vi "MultiChannelExample.vi"() -> ()   [LabVIEW 2020]
uses:
  PalmSens/PalmSens.lvclass
  D:/PalmSensAppsAndSDKS/LabVIEW/PalmSens SDK for LabVIEW 5.10/PalmSens/Libraries/PalmSens.Core.dll
  PalmSens/Libraries/PalmSens.Core.dll
  PalmSens/MeasurementsResult.ctl
  PalmSens/MeasurementResults.ctl
  PalmSens/LiveCurveResult.ctl
panel:
  out "Measurements":T1
  out "Array 2":string[](array[string])
  out "Is Measuring 2":bool
  in  "PalmSens.lvclass 2":refnum<class "PalmSens.lvclass">
  out "LSV Method Indicator":refnum<k24>
  out "Array":string[](array[string])
  out "Is Measuring":bool
  in  "PalmSens.lvclass":refnum<class "PalmSens.lvclass">
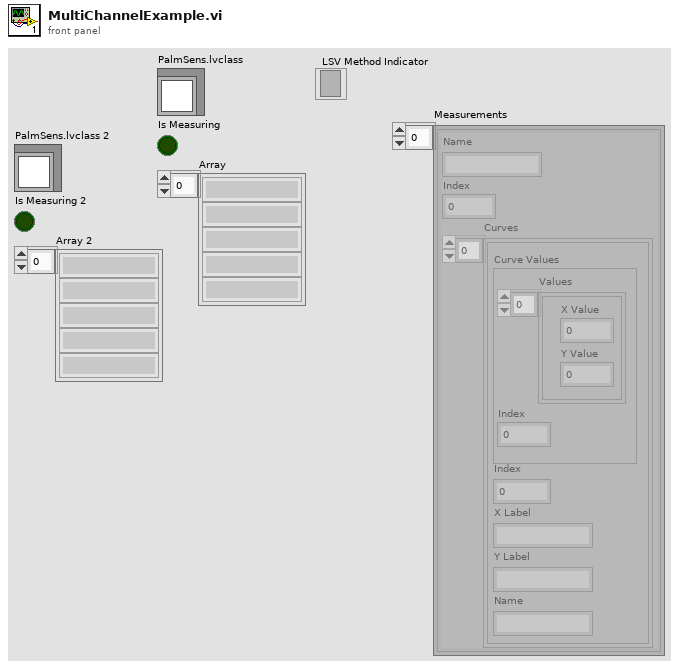
[diagram p1: front panel]
types:
  T1 = typedef "MeasurementsResult.ctl" = cluster{"Name":string, "Curves":T2, "Index":i32}[]
  T2 = typedef "MeasurementResults.ctl" = T3[]
  T3 = typedef "LiveCurveResult.ctl" = cluster{"X Label":string, "Y Label":string, "Name":string, "Index":i16, "Curve Values":cluster{"Values":cluster{"X Value":dbl, "Y Value":dbl}[], "Index":i16}}
  T4 = cluster{"Active Measurement":refnum<k24>, "Is Measuring Refnum":refnum<vi>, "Live Curve Result Refnum":refnum<vi>}
  T5 = cluster{"Active Measurement":refnum<k24>, "Is Measuring Refnum":refnum<vi>, "Live Curve Result Refnum":refnum<vi>}[]
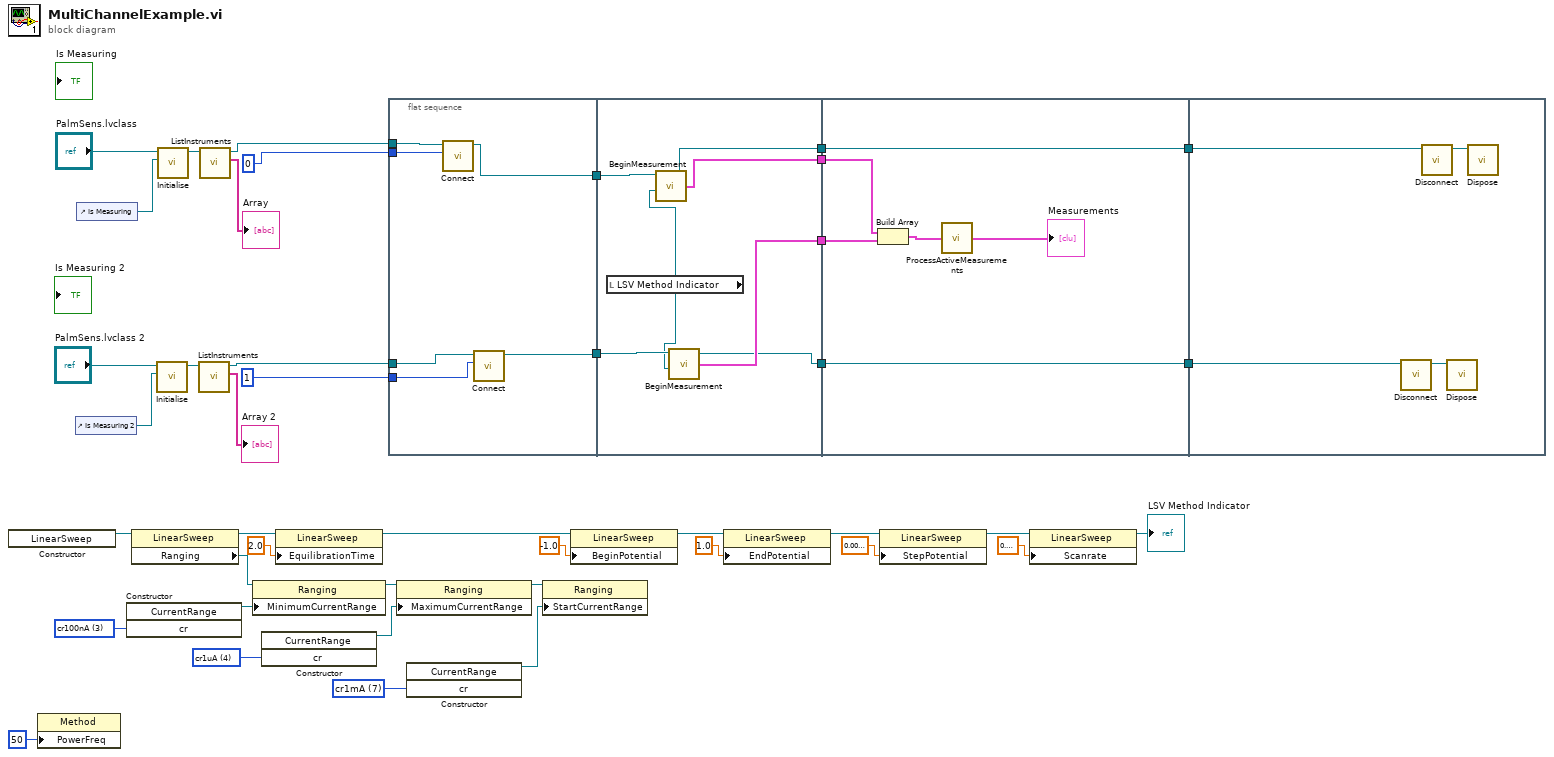
[diagram p0: block diagram]
diagram:
  w31 = 4 items=["cr100pA"=0, "cr1nA"=1, "cr10nA"=2, "cr100nA"=3, "cr1uA"=4, "cr10uA"=5, "cr100uA"=6, "cr1mA"=7, "cr10mA"=8, "cr100mA"=9, "cr2uA"=10, "cr4uA"=11, "cr8uA"=12, "cr16uA"=13, "cr32uA"=14, "cr125uA"=17, "cr250uA"=18, "cr500uA"=19, "cr5mA"=20, "cr6uA"=21, "cr13uA"=22, "cr25uA"=23, "cr50uA"=24, "cr200uA"=25, "cr63uA"=26] ("cr")
  w32 = 7 items=["cr100pA"=0, "cr1nA"=1, "cr10nA"=2, "cr100nA"=3, "cr1uA"=4, "cr10uA"=5, "cr100uA"=6, "cr1mA"=7, "cr10mA"=8, "cr100mA"=9, "cr2uA"=10, "cr4uA"=11, "cr8uA"=12, "cr16uA"=13, "cr32uA"=14, "cr125uA"=17, "cr250uA"=18, "cr500uA"=19, "cr5mA"=20, "cr6uA"=21, "cr13uA"=22, "cr25uA"=23, "cr50uA"=24, "cr200uA"=25, "cr63uA"=26] ("cr")
  w36 = 3 items=["cr100pA"=0, "cr1nA"=1, "cr10nA"=2, "cr100nA"=3, "cr1uA"=4, "cr10uA"=5, "cr100uA"=6, "cr1mA"=7, "cr10mA"=8, "cr100mA"=9, "cr2uA"=10, "cr4uA"=11, "cr8uA"=12, "cr16uA"=13, "cr32uA"=14, "cr125uA"=17, "cr250uA"=18, "cr500uA"=19, "cr5mA"=20, "cr6uA"=21, "cr13uA"=22, "cr25uA"=23, "cr50uA"=24, "cr200uA"=25, "cr63uA"=26] ("cr")
  n1 = constructor class="LinearSweep"() -> (reference out=w38:refnum<k24>)  [unwired: 3 in, 2 out]
  n2 = property class="Method"("PowerFreq"=50) -> ()  [unwired: 2 in, 2 out]
  n3 = control-ref of="Is Measuring 2"() -> (w15:refnum<vi>)
  n4 = control-ref of="Is Measuring"() -> (w41:refnum<vi>)
  n5 = constructor class="CurrentRange"("cr"=w36) -> (reference out=w35:refnum<k24>)  [unwired: 3 in, 3 out]
  n6 = property class="LinearSweep"(reference=w38) -> (reference out=w28:refnum<k24>, "Ranging"=w37:refnum<k24>)  [unwired: 1 in, 1 out]
  n7 = call-dynamic "Initialise.vi"("Is Measuring Refnum"=w15, "PalmSens in"="PalmSens.lvclass 2") -> ("PalmSens out"=w14:refnum<class "PalmSens.lvclass">)  [unwired: 8 in, 1 out]
  n8 = call-dynamic "Initialise.vi"("Is Measuring Refnum"=w41, "PalmSens in"="PalmSens.lvclass") -> ("PalmSens out"=w40:refnum<class "PalmSens.lvclass">)  [unwired: 8 in, 1 out]
  n9 = call-dynamic "ListInstruments.vi"("PalmSens in"=w14) -> ("Array"=→"Array 2":string[], "PalmSens out"=w1:refnum<class "PalmSens.lvclass">)  [unwired: 8 in, 1 out]
  n10 = call-dynamic "ListInstruments.vi"("PalmSens in"=w40) -> ("Array"=→"Array":string[], "PalmSens out"=w3:refnum<class "PalmSens.lvclass">)  [unwired: 8 in, 1 out]
  n11 = property class="Ranging"(reference=w37, "MinimumCurrentRange"=w35) -> (reference out=w34:refnum<k24>)  [unwired: 1 in, 1 out]
  n12 = constructor class="CurrentRange"("cr"=w31) -> (reference out=w29:refnum<k24>)  [unwired: 3 in, 3 out]
  n13 = property class="LinearSweep"(reference=w28, "EquilibrationTime"=sgl 2.0) -> (reference out=w26:refnum<k24>)  [unwired: 1 in, 1 out]
  n14 = flat-sequence {
    tunnel: [w46] -> w6
    tunnel: [w43] -> w5
    tunnel: 0 ("Instrument Index") -> [w48]
    tunnel: w3 -> [w47]
    tunnel: 1 ("Instrument Index") -> [w45]
    tunnel: w1 -> [w44]
    tunnel: [w53] -> w10
    tunnel: [w50] -> w9
    tunnel: [w54] -> w8
    tunnel: [w51] -> w7
    tunnel: w6 -> [w55]
    tunnel: w5 -> [w52]
    tunnel: [w61] -> w12
    tunnel: [w60] -> w11
    tunnel: w10 -> [w61]
    tunnel: w9 -> [w60]
    tunnel: w8 -> [w59]
    tunnel: w7 -> [w58]
    tunnel: w12 -> [w63]
    tunnel: w11 -> [w62]
    frame #0 {
      n15 = call-dynamic "Connect.vi"("Instrument Index"=w48, "PalmSens in"=w47) -> ("PalmSens out"=w46:refnum<class "PalmSens.lvclass">)  [unwired: 8 in, 1 out]
      n16 = call-dynamic "Connect.vi"("Instrument Index"=w45, "PalmSens in"=w44) -> ("PalmSens out"=w43:refnum<class "PalmSens.lvclass">)  [unwired: 8 in, 1 out]
    }
    frame #1 {
      n17 = local read "LSV Method Indicator"() -> (w49:refnum<k24>)
      n18 = call-dynamic "BeginMeasurement.vi"("Method .NET Refnum"=w49, "PalmSens in"=w55) -> ("Active Measurement Info"=w54:T4, "PalmSens out"=w53:refnum<class "PalmSens.lvclass">)  [unwired: 2 in, 1 out]
      n19 = call-dynamic "BeginMeasurement.vi"("Method .NET Refnum"=w49, "PalmSens in"=w52) -> ("Active Measurement Info"=w51:T4, "PalmSens out"=w50:refnum<class "PalmSens.lvclass">)  [unwired: 2 in, 1 out]
    }
    frame #2 {
      n20 = Build Array(w59, w58) -> (w57:T5)
      n21 = call "ProcessActiveMeasurements.vi"("Active Measurements"=w57) -> ("Measurements"=→"Measurements":T1)
    }
    frame #3 {
      n22 = call-dynamic "Disconnect.vi"("PalmSens in"=w62) -> ("PalmSens out"=w64:refnum<class "PalmSens.lvclass">)  [unwired: 9 in, 1 out]
      n23 = call-dynamic "Disconnect.vi"("PalmSens in"=w63) -> ("PalmSens out"=w65:refnum<class "PalmSens.lvclass">)  [unwired: 9 in, 1 out]
      n24 = call-dynamic "Dispose.vi"("PalmSens in"=w64) -> ()  [unwired: 9 in, 2 out]
      n25 = call-dynamic "Dispose.vi"("PalmSens in"=w65) -> ()  [unwired: 9 in, 2 out]
    }
  }
  n26 = property class="Ranging"(reference=w34, "MaximumCurrentRange"=w29) -> (reference out=w33:refnum<k24>)  [unwired: 1 in, 1 out]
  n27 = constructor class="CurrentRange"("cr"=w32) -> (reference out=w30:refnum<k24>)  [unwired: 3 in, 3 out]
  n28 = property class="Ranging"(reference=w33, "StartCurrentRange"=w30) -> ()  [unwired: 1 in, 2 out]
  n29 = property class="LinearSweep"(reference=w26, "BeginPotential"=sgl -1.0) -> (reference out=w24:refnum<k24>)  [unwired: 1 in, 1 out]
  n30 = property class="LinearSweep"(reference=w24, "EndPotential"=sgl 1.0) -> (reference out=w22:refnum<k24>)  [unwired: 1 in, 1 out]
  n31 = property class="LinearSweep"(reference=w22, "StepPotential"=sgl 0.01) -> (reference out=w20:refnum<k24>)  [unwired: 1 in, 1 out]
  n32 = property class="LinearSweep"(reference=w20, "Scanrate"=sgl 0.2) -> (reference out=→"LSV Method Indicator":refnum<k24>)  [unwired: 1 in, 1 out]
